vi "ExSubCollectDisplayStoreCoolSnap_test.vi"(3 "error in (no error)":errorcluster, 4 "Store flag":i8, 6 "Handle Cluster":T1) -> (0 "error out":errorcluster, 1 "got frame":u32, 2 "Handle Cluster Out":T1)   [LabVIEW 2015]
panel:
  # "ExSubCollectDisplayStoreCoolSnap:\nThis sub-VI checks to see if data has arrived from camera,\nif so it then puts it in image object and displays it. If store \nswitch is set it will also store it."
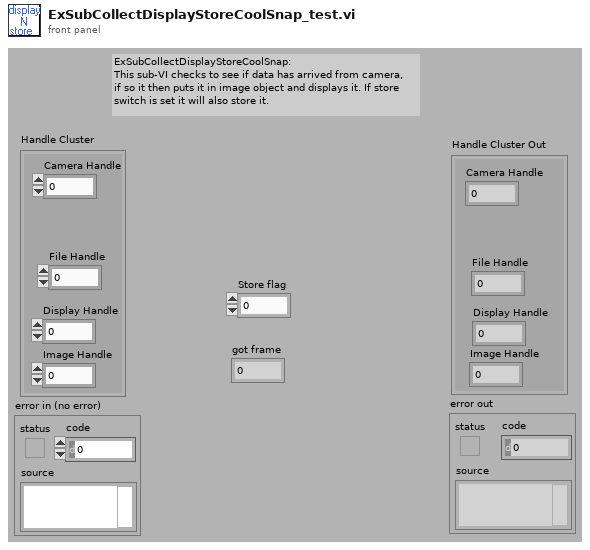
[diagram p1: front panel]
types:
  T1 = cluster{"Camera Handle":u32, "File Handle":u32, "Display Handle":u32, "Image Handle":u32}
  T2 = cluster{"Camera Handle":u32, "File Handle":u32, "Display Handle":u32, "Data Handle":u32}
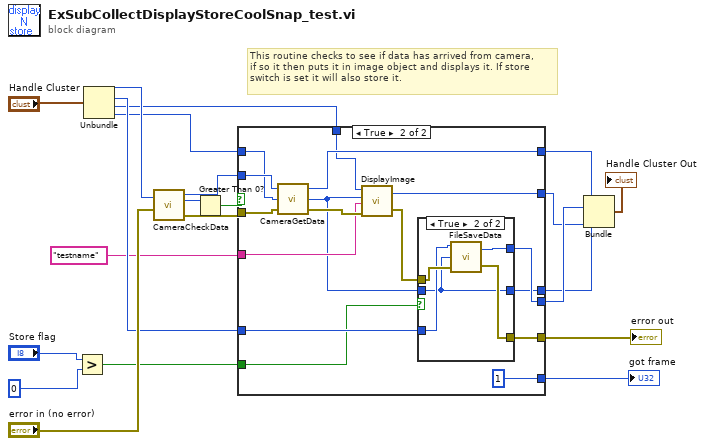
[diagram p0: block diagram]
diagram:
  # "This routine checks to see if data has arrived from camera,\nif so it then puts it in image object and displays it. If store \nswitch is set it will also store it."
  n1 = Greater?(x="Store flag", y=0) -> (0:w6:bool)
  n2 = Unbundle("Handle Cluster") -> ("Camera Handle"=w12:u32, "File Handle"=w4:u32, "Display Handle"=w3:u32, "Image Handle"=w2:u32)
  n3 = call <userlib>:"CameraCheckData.vi"("Camera Handle"=w12, "error in"="error in (no error)") -> ("Camera Handle"=w18:u32, "Number Of Frames Available"=w17:i32, "error out"=w16:errorcluster)
  n4 = Greater Than 0?(x=w17) -> (x > 0?=w19:bool)
  n5 = case shown="True" w19 {
    tunnel: w18 -> [w27 w43]
    tunnel: w16 -> [w26 w42]
    tunnel: w2 -> [w23 w37]
    tunnel: w3 -> [w25 w36]
    tunnel: [w27 w41] -> w13
    tunnel: [w24 w40] -> w11
    tunnel: "testname" -> [_ w35]
    tunnel: w4 -> [w24 w34]
    tunnel: [w25 w33] -> w10
    tunnel: [w26 w32] -> w14
    tunnel: [w23 w30] -> w9
    tunnel: w6 -> [_ w29]
    tunnel: [0 1] -> w5
    frame False {
    }
    frame True {
      n6 = call <userlib>:"CameraGetData.vi"("error in"=w42, "Data Handle"=w37, "Camera Handle"=w43) -> ("error out"=w39:errorcluster, "Data Handle"=w31:u32, "Camera Handle"=w41:u32)
      n7 = call <userlib>:"DisplayImage.vi"("error in"=w39, "Title"=w35, "Image Handle"=w31, "Display Handle"=w36) -> ("error out"=w38:errorcluster, "Display Handle"=w33:u32)
      n8 = case shown="True" w29 {
        tunnel: [w46 w51] -> w40
        tunnel: w38 -> [w45 w50]
        tunnel: w34 -> [w46 w48]
        tunnel: [w45 w49] -> w32
        tunnel: w31 -> [w44 w47]
        tunnel: [w44 w47] -> w30
        frame False {
        }
        frame True {
          n9 = call <userlib>:"FileSaveData.vi"("error in"=w50, "Image Handle"=w47, "File Handle"=w48) -> ("error out"=w49:errorcluster, "File Handle"=w51:u32)
        }
      }
    }
  }
  "error out" <- w14
  "got frame" <- w5
  n10 = Bundle("Camera Handle"=w13, "File Handle"=w11, "Display Handle"=w10, "Data Handle"=w9) -> (→"Handle Cluster Out":T2)  [unwired: 1 in]
